vi "sensor config set label.vi"(9 "str_length":i32, 10 "label_str":string, 11 "device_handle":u32) -> (2 "function return":i32, 3 "device_handle out":u32)   [LabVIEW 2019, in "apdm.lvlib"]
doc: "APDM_EXPORT int apdm_sensor_config_set_label(apdm_device_handle_t device_handle, const char label_str[16], const int str_length);"
uses:
  apdm.lvlib
  Lee Lab/CP FES Walking 2018/Code/Working/LabVIEW/apdm.dll
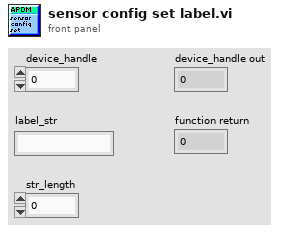
[diagram p1: front panel]
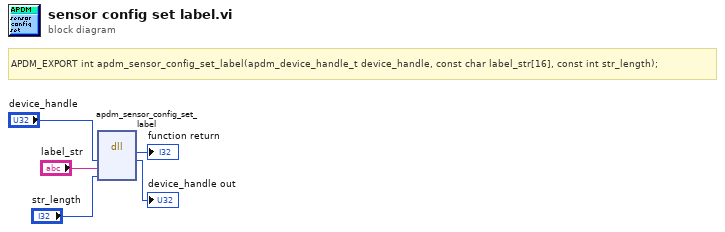
[diagram p0: block diagram]
diagram:
  # "APDM_EXPORT int apdm_sensor_config_set_label(apdm_device_handle_t device_handle, const char label_str[16], const int str_length);"
  n1 = dll-call lib="C:/Users/jfalesi/Dropbox/Lee Lab/CP FES Walking 2018/Code/Working/LabVIEW/apdm.*" fn="apdm_sensor_config_set_label"("device_handle"="device_handle", "label_str"="label_str", "str_length"="str_length") -> (→"function return":i32, "device_handle"=→"device_handle out":u32)  [unwired: 5 in, 2 out]
